vi "Go to Guide.vi"(8 "error in (no error)":errorcluster, 11 "States.lvlib:Guide.lvclass":refnum<class "Guide.lvclass">) -> (0 "error out":errorcluster, 3 "Process State out":refnum<class "State Actor.lvclass">)   [LabVIEW 2014, in "States.lvlib" / "Guide.lvclass"]
uses:
  Guide.lvclass
  <vilib>/NI/Actors/State Actor/State Actor/State Actor.lvclass
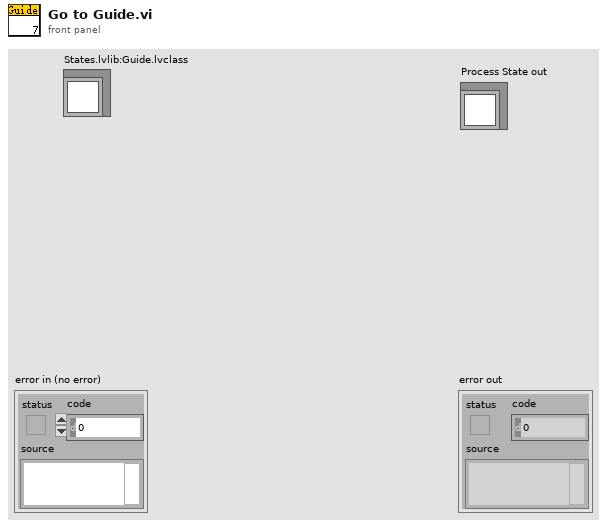
[diagram p1: front panel]
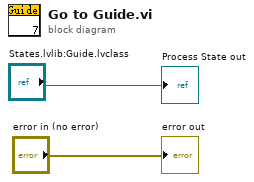
[diagram p0: block diagram]
diagram:
  "error out" <- "error in (no error)"
  "Process State out" <- "States.lvlib:Guide.lvclass"
